vi "Actor Core.vi"(8 "error in":errorcluster, 11 "Nested in":refnum<class "Top.lvclass">) -> (0 "error out":errorcluster, 3 "Actor out":refnum<class "Actor.lvclass">)   [LabVIEW 2021, in "Top.lvlib" / "Top.lvclass"]
doc: "(<B>Filename</B>: Actor Framework.lvlib:Actor.lvclass:Actor Core.vi)\n\nReceives messages to the actor, reacts to them, and initiates any error handling that may shut the actor down.\n\nDescendant classes may override this VI to append parallel tasks for the actor to complete while it handles messages. Overrides use the Call Parent Method node."
uses:
  Top.lvclass
  C:/Program Files/National Instruments/LabVIEW 2021/vi.lib/MGI/Panel Manager/Panel Actor/Panel Actor/Panel Actor.lvclass
  C:/Program Files/National Instruments/LabVIEW 2021/vi.lib/ActorFramework/Actor/Actor.lvclass
  <vilib>/ActorFramework/Actor/Actor.lvclass
  Service/Service.lvclass
  <vilib>/ActorFramework/Actor/Actor.lvclass/Actor.ctl
  <vilib>/ActorFramework/Message Enqueuer/Message Enqueuer.lvclass/Message Enqueuer.ctl
  Top.lvclass/Top.ctl
  Top Messages/Password Authentication Msg/Password Authentication Msg.lvclass/Password Authentication Msg.ctl
  <vilib>/ActorFramework/Message Enqueuer/Init from Existing Queue.vi
  <vilib>/ActorFramework/Message Enqueuer/Enqueue.vi
  <vilib>/MGI/Panel Manager/Panel/Panel/Window/Window.lvclass
  C:/Program Files/National Instruments/LabVIEW 2021/vi.lib/MGI/Panel Manager/Panel/Panel/Panel.lvclass
  Top Messages/Password Authentication Msg/Password Authentication Msg.lvclass
  C:/Program Files/National Instruments/LabVIEW 2021/vi.lib/ActorFramework/Message/Message.lvclass
  <vilib>/ActorFramework/Stop Msg/Stop Msg.lvclass
  <vilib>/ActorFramework/Message Priority Queue/Priority Enqueue.vi
  <vilib>/MGI/Panel Manager/Panel/Panel/Window/Window.vi
  <vilib>/ActorFramework/Message Enqueuer/Message Enqueuer.lvclass
  <vilib>/MGI/Panel Manager/Panel Actor/Panel Actor/Panel Actor.lvclass
  C:/git/IV-Curve-PH316/Source/Top/Top.lvclass
  <vilib>/MGI/Panel Manager/Panel/Panel.lvlib
  C:/git/IV-Curve-PH316/Source/Service/Service.lvclass
  C:/Program Files/National Instruments/LabVIEW 2021/vi.lib/MGI/Panel Manager/Panel/Panel/Window/Window.lvclass
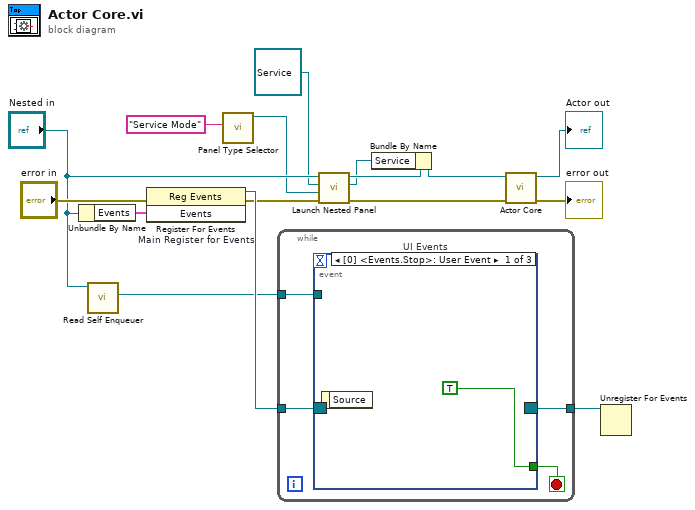
[diagram p0: block diagram]
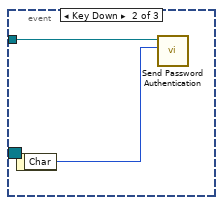
[diagram p2: hidden frame]
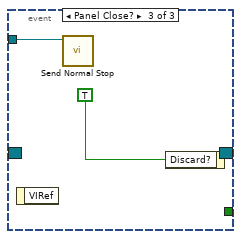
[diagram p3: hidden frame]
diagram:
  n1 = Unbundle By Name("Nested in") -> ("Events"=w14:cluster{"Stop":refnum<user-event>})
  n2 = call <vilib>:"Read Self Enqueuer.vi"("Actor"="Nested in") -> ("Self Enqueuer"=w12:refnum<class "Message Enqueuer.lvclass">)  [unwired: 10 in]
  n3 = register-events "Main Register for Events"(error in="error in", w14) -> (reference out=w15:refnum<event-registration>, error out=w7:errorcluster)  [unwired: 1 in]
  n4 = call-poly <vilib>:"Panel Type Selector.vi"("Default Title"="Service Mode") -> ("Window out"=w5:refnum<class "Window.lvclass">)  [unwired: 9 in, 1 out]
  n5 = while {
    tunnel: w15 -> [w20]
    tunnel: [w18] -> w13
    tunnel: w12 -> [w17]
    stop <- w19 stop-if-true
    n6 = event "UI Events" shown="[0] <Events.Stop>: User Event" {
      selector: w20 -> [_ _ _]
      dyn-events: [_ _ _] -> w18
      timeout: _ -> [_ _ _]
      tunnel: [TRUE _ _] -> w19
      tunnel: w17 -> [_ w23 w24]
      event User Event {
        n7 = event-data() -> ()  [unwired: 1 in, 1 out]
      }
      event Key Down {
        n8 = event-data() -> ("Char"=w22:i16)  [unwired: 1 in]
        n9 = call "Send Password Authentication.vi"("Key"=w22, "Message Enqueuer"=w23) -> ()  [unwired: 8 in, 2 out]
      }
      event Panel Close? {
        n10 = event-data() -> ()  [unwired: 1 in, 1 out]
        n11 = call <vilib>:"Send Normal Stop.vi"("Message Enqueuer"=w24) -> ()  [unwired: 10 in, 1 out]
        n12 = event-data("Discard?"=TRUE) -> ()  [unwired: 1 in, 1 out]
      }
    }
  }
  n13 = call <vilib>:"Launch Nested Panel.vi"("error in (no error)"=w7, "Panel"=w5, "Nested Panel Actor"=refnum<class "Service.lvclass"> refnum ("Service.lvlib:Service.lvclass"), "Panel Actor in"="Nested in") -> ("error out"=w6:errorcluster, "Nested Actor's Enqueuer"=w2:refnum<class "Message Enqueuer.lvclass">, "Panel Actor out"=w8:refnum<class "Top.lvclass">)  [unwired: 4 in, 1 out]
  n14 = Bundle By Name(cluster=w8, "Service"=w2) -> (w3:refnum<class "Top.lvclass">)
  n15 = call-parent "Actor Core.vi"("error in"=w6, "Panel Actor in"=w3) -> ("error out"=→"error out":errorcluster, "Actor out"=→"Actor out":refnum<class "Actor.lvclass">)  [unwired: 8 in]
  n16 = Unregister For Events(event registration refnum=w13) -> ()  [unwired: 1 in, 1 out]
